vi "输出停止.vi"(4 "启动项":u16(ring) items=["电压停止", "电流停止", "全部停止", "UB_outPut_stop", "IB_outPut_stop", "UC_outPut_stop"], 5 "串口号":refnum<visa-resource-name>) -> (1 "应答":string)   [LabVIEW 2014]
panel:
  in  "数据":u16[](array[numeric]) format="%.0x"
  in  "数据标识":u8[](array[numeric]) format="%.0x"
  in  "长度":i32
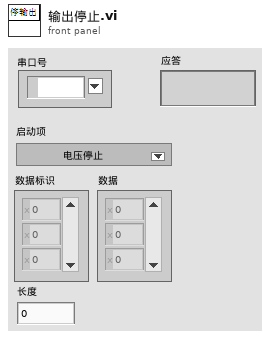
[diagram p1: front panel]
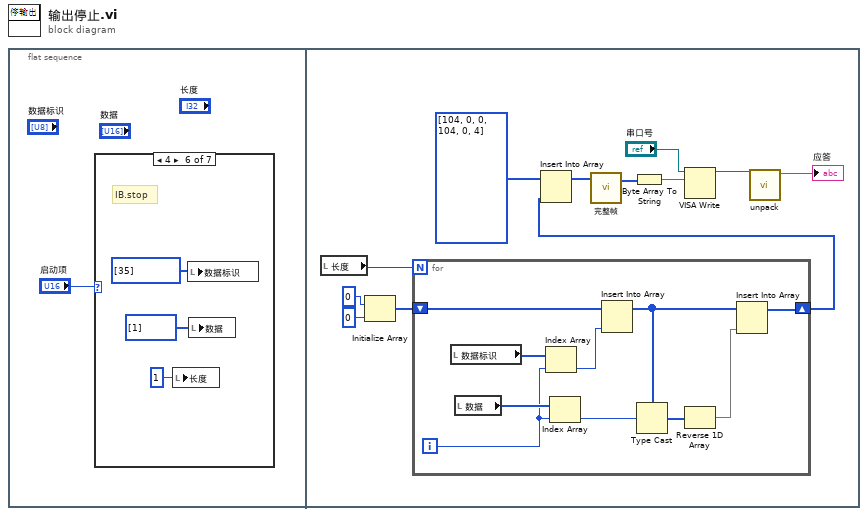
[diagram p0: block diagram]
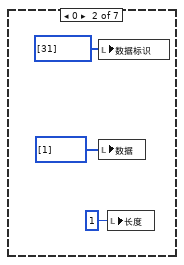
[diagram p3: hidden frame]
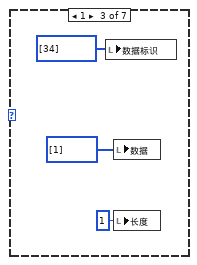
[diagram p4: hidden frame]
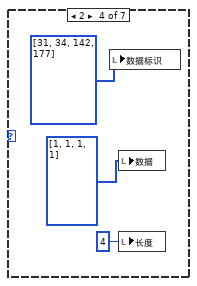
[diagram p5: hidden frame]
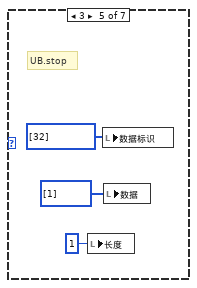
[diagram p6: hidden frame]
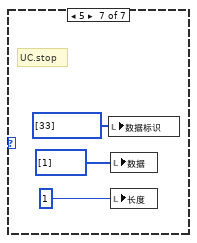
[diagram p7: hidden frame]
diagram:
  n1 = flat-sequence {
    frame #0 {
      n2 = case shown="4" "启动项" {
        frame Default {
        }
        frame 0 {
          n3 = local write "数据标识"(u8[] [31] ("数据标识")) -> ()
          n4 = local write "数据"(u16[] [1] ("数据标识")) -> ()
          n5 = local write "长度"(1 ("长度")) -> ()
        }
        frame 1 {
          n6 = local write "数据标识"(u8[] [34] ("数据标识")) -> ()
          n7 = local write "数据"(u16[] [1] ("数据标识")) -> ()
          n8 = local write "长度"(1 ("长度")) -> ()
        }
        frame 2 {
          n9 = local write "数据标识"(u8[] [31, 34, 142, 177] ("数据标识")) -> ()
          n10 = local write "数据"(u16[] [1, 1, 1, 1] ("数据标识")) -> ()
          n11 = local write "长度"(4 ("长度")) -> ()
        }
        frame 3 {
          # "UB.stop"
          n12 = local write "长度"(1 ("长度")) -> ()
          n13 = local write "数据标识"(u8[] [32] ("数据标识")) -> ()
          n14 = local write "数据"(u16[] [1] ("数据标识")) -> ()
        }
        frame 4 {
          # "IB.stop"
          n15 = local write "长度"(1 ("长度")) -> ()
          n16 = local write "数据标识"(u8[] [35] ("数据标识")) -> ()
          n17 = local write "数据"(u16[] [1] ("数据标识")) -> ()
        }
        frame 5 {
          # "UC.stop"
          n18 = local write "数据标识"(u8[] [33] ("数据标识")) -> ()
          n19 = local write "数据"(u16[] [1] ("数据标识")) -> ()
          n20 = local write "长度"(1 ("长度")) -> ()
        }
      }
    }
    frame #1 {
      n21 = local read "长度"() -> (w26:i32)
      n22 = Initialize Array(u8 0 ("元素"), 0 ("维数大小")) -> (w30:u8[])
      n23 = for {
        N: w26 -> [_]
        shift-right: [w32] -> w27
        shift-left: w30 -> [w38]
        i -> [w39]
        n24 = local read "数据标识"() -> (w41:u8[])
        n25 = local read "数据"() -> (w40:u16[])
        n26 = Index Array(array=w41, index=w39) -> (element=w37:u8)
        n27 = Index Array(array=w40, index=w39) -> (element=w34:u16)
        n28 = Insert Into Array(array=w38, new element=w37) -> (w35:u8[])  [unwired: 1 in]
        n29 = Type Cast(type=w35, x=w34) -> (*(type *) &x=w36:u8[])
        n30 = Reverse 1D Array(array=w36) -> (reversed array=w33:u8[])
        n31 = Insert Into Array(array=w35, new element=w33) -> (w32:u8[])  [unwired: 1 in]
      }
      n32 = Insert Into Array(array=u8[] [104, 0, 0, 104, 0, 4], new element=w27) -> (w25:u8[])  [unwired: 1 in]
      n33 = call "完整帧.vi"("不完整帧"=w25) -> ("完整帧"=w20:u8[])  [unwired: 2 in]
      n34 = Byte Array To String(unsigned byte array=w20) -> (string=w21:string)
      n35 = VISA Write(VISA resource name="串口号", write buffer=w21) -> (VISA resource name out=w23:refnum<visa-resource-name>)  [unwired: 1 in, 2 out]
      n36 = call "unpack.vi"("串口号输入"=w23) -> ("应答"=→"应答":string)  [unwired: 5 in, 1 out]
    }
  }
